vi "Negate_Qin.vi"(8 "valid in":bool, 11 "Data in":fxp<+/-,16,14>[](array[numeric])=[0.0, 0.0, 0.0, 0.0]) -> (0 "valid out":bool, 3 "Data out":fxp<+/-,16,14>[](array[numeric]))   [LabVIEW 2013]
uses:
  <vilib>/rvi/FXPMathLib/FxpConvert/subVIs/nifxpmath_Convert_SimConfig.ctl
  <vilib>/fxp/LVFixedPointQuantizationPolicyTypeDef.ctl
  <vilib>/fxp/LVFixedPointOverflowPolicyTypeDef.ctl
  <vilib>/rvi/FXPMathLib/FxpConvert/simVIs/DllFxpConvertTemp_sub.vi
  <vilib>/rvi/FXPMathLib/FxpConvert/XNode/nifxpmath_Convert.xnode
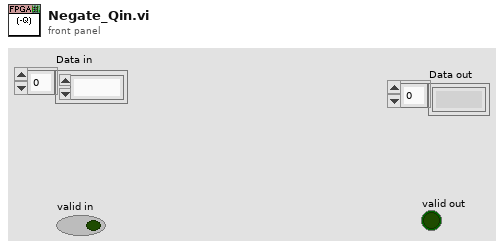
[diagram p1: front panel]
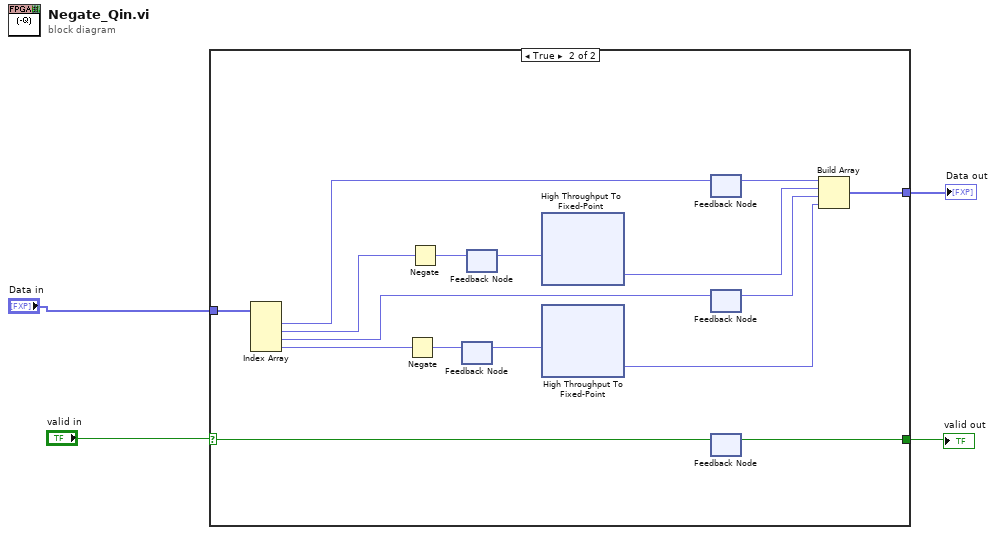
[diagram p0: block diagram]
diagram:
  n1 = case shown="True" "valid in" {
    selector: "valid in" -> [w5 w18]
    tunnel: "Data in" -> [w6 w22]
    tunnel: [w5 w19] -> w3
    tunnel: [w6 w11] -> w1
    frame False {
    }
    frame True {
      n2 = Index Array(array=w22) -> (element #1=w17:fxp<+/-,16,14>, element #2=w16:fxp<+/-,16,14>, element #3=w12:fxp<+/-,16,14>, element #4=w14:fxp<+/-,16,14>)  [unwired: 4 in]
      n3 = Negate(x=w14) -> (-x=w13:fxp<+/-,17,15>)
      n4 = Negate(x=w16) -> (-x=w15:fxp<+/-,17,15>)
      n5 = feedback #1() -> (w10:fxp<+/-,17,15>)  [unwired: 1 in]
      n6 = feedback-in #1(w13) -> ()
      n7 = feedback #2() -> (w7:fxp<+/-,17,15>)  [unwired: 1 in]
      n8 = feedback-in #2(w15) -> ()
      n9 = xnode "High Throughput To Fixed-Point"("x"=w7) -> ("y"=w8:fxp<+/-,16,14>)
      n10 = xnode "High Throughput To Fixed-Point"("x"=w10) -> ("y"=w9:fxp<+/-,16,14>)
      n11 = feedback #3() -> (w21:fxp<+/-,16,14>)  [unwired: 1 in]
      n12 = feedback-in #3(w17) -> ()
      n13 = feedback #4() -> (w20:fxp<+/-,16,14>)  [unwired: 1 in]
      n14 = feedback-in #4(w12) -> ()
      n15 = feedback #5() -> (w19:bool)  [unwired: 1 in]
      n16 = feedback-in #5(w18) -> ()
      n17 = Build Array(w21, w8, w20, w9) -> (w11:fxp<+/-,16,14>[])
    }
  }
  "valid out" <- w3
  "Data out" <- w1
